vi "7.vi"(11 "Unit (0: Celsius)":enum16{"Fahrenheit", "Celsius"}(ring)) -> (3 "Temperature Value":dbl(slide) scale=0.0..10.0)   [LabVIEW 2015]
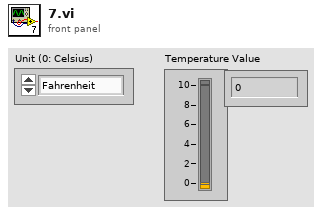
[diagram p1: front panel]
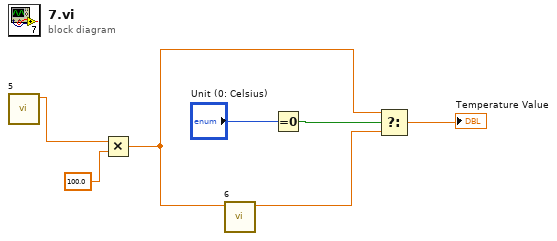
[diagram p0: block diagram]
diagram:
  n1 = call "5.vi"() -> ("Voltage"=w2:dbl)  [unwired: 10 in, 1 out]
  n2 = Multiply(x=w2, y=100.0) -> (x*y=w5:dbl)
  n3 = call "6.vi"("Degrees Celcius"=w5) -> ("Degrees Fahrenheit"=w6:dbl)  [unwired: 10 in]
  n4 = Equal To 0?(x="Unit (0: Celsius)") -> (x = 0?=w7:bool)
  n5 = Select(t=w5, s=w7, f=w6) -> (s? t:f=→"Temperature Value":dbl)
